vi "Save DataBuffer.vi"(0 "File Parameter":T8={"Filename Prefix"="MyData", "Extension"=enum."±Field", "Suffix"="", "Current Path"=path "/opticsmac/Users/Data"}, 7 "User Comments":string="This data's for you!\nType \u0011-H to get a help window for the various controls.", 13 "FileFormat":T7={"File Format"=enum."Macintosh (EOL: CR)", "Delimiter"=enum."TAB", "SaveComments?"=enum."Saved in the Header Area"}) -> (4 "File Info output":T1={"FilePath"=path "/DATA/Labview Items", "Field (T)"=55.0, "Temperature (K)"=77.0, "X-Axis"=enum."nm", "Center nm"=55.0, "Current Grating Density"=enum."600", "CCD Parameters"={"Exposure Time (s)"=0.2, "Offset"=0.0, "BkgrdCrct"=FALSE, "Shutter"=FALSE, "Mode"=enum."Regular", "Repetition"=4, "dt or s"=0.0}, "Operation Mode"=enum."NML Data Acquisition", "Exp Index"=0, "Index_repetition"=0, "Index"=0, "Current Detector"=enum."CCD-1024x256"} {"CCD Parameters"."dt or s" format="%#.6f"; "CCD Parameters"."Repetition" min=1; "CCD Parameters"."Offset" format="%#.2f"; "CCD Parameters"."Exposure Time (s)" min=0.02 max=6000.0 format="%#.2f"; "Center nm" format="%.2f"; "Temperature (K)" format="%.2f"; "Field (T)" format="%.2f"})   [LabVIEW 2019]
doc: "Write (FIFO) or retrieve (LIFO) data from the buffer.\n\nWhen write to the buffer, set the desired \"Buffer Size\" and run the VI several iterations. Notice that initially, the buffer grows to reach \"Buffer Size\" and then the input data flows from the last buffer element through to the zero element on each iteration (First In, First Out).\n\nWhen read from the buffer, set the Read# to the nth previous input data, i.e. counting reversely, with the most recent input counted as the 1st readout. If the input is out of current buffer size, an error is returned. (Last In, First Out)"
uses:
  Globals and TypeDefs/Type Definitions.llb/FilePathParameter.ctt
  Globals and TypeDefs/Type Definitions.llb/FileFormatParameter.ctt
  Globals and TypeDefs/Type Definitions.llb/FileInfoParameter.ctt
  Globals and TypeDefs/Type Definitions.llb/Wavelength Unit.ctt
  Globals and TypeDefs/Type Definitions.llb/McPherson Grating Density.ctl
  Globals and TypeDefs/Type Definitions.llb/CCDParameter.ctt
  Globals and TypeDefs/Type Definitions.llb/OperationMode.ctt
  Globals and TypeDefs/Type Definitions.llb/ListOfDetectors.ctt
  File and save/X-Axis_Generator_morph.vi
panel:
  out "X-Axis":i32(ring)=1 items=["Point #", "nm", "eV", "meV", "cm-1"]
  in  "continue2":bool=TRUE
  in  "Speed":u16(slide)=100 min=50 max=5000 step=50 scale=10.0..5000.0
  in  "Movie":bool
  out "Continue?":bool
  out "File Contents":string
  in  "WL unit":i32(ring)=1 items=["Wavelength", "nm", "eV", "meV", "cm-1"]
  in  "Save":bool
  in  "Cancel":bool
  out "File Path":path
  out "?":T9(graph)
  in  "Read#":u16(slide)=1 min=1 max=27 step=1 scale=1.0..27.0
  # "Latest"
  # "Erliest"
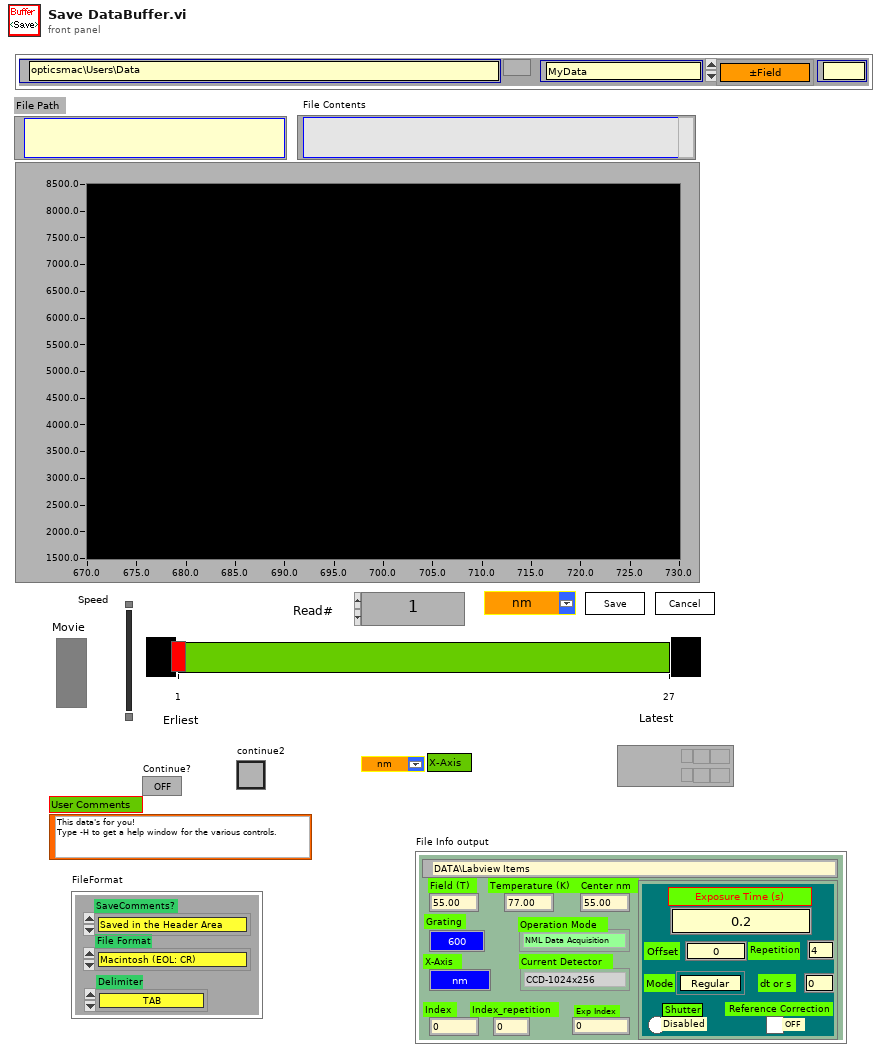
[diagram p1: front panel]
types:
  T1 = typedef "FileInfoParameter.ctt" = cluster{"FilePath":path, "Field (T)":dbl, "Temperature (K)":dbl, "X-Axis":T2, "Center nm":dbl, "Current Grating Density":T3, "CCD Parameters":T4, "Operation Mode":T5, "Exp Index":u32, "Index_repetition":u16, "Index":u16, "Current Detector":T6}
  T2 = typedef "Wavelength Unit.ctt" = enum8{"Point", "nm", "eV", "meV", "cm_1"}
  T3 = typedef "McPherson Grating Density.ctl" = enum8{"150", "300", "600", "1200", "1800"}
  T4 = typedef "CCDParameter.ctt" = cluster{"Exposure Time (s)":dbl, "Offset":dbl, "BkgrdCrct":bool, "Shutter":bool, "Mode":enum8{"Regular", "OverExp Cor", "SpikeRemove", "ForCalibration"}, "Repetition":u16, "dt or s":dbl}
  T5 = typedef "OperationMode.ctt" = enum16{"Standby", "CCD Single Shot", "CCD Sequence Shots", "CCD Custom Shots", "CCD Reference Shot", "Step Scanning ", "Time Scanning", "NML Data Acquisition"}
  T6 = typedef "ListOfDetectors.ctt" = enum8{"CCD-1024x256", "InGaAs PDA-1024x1", "CCD-1340x400", "Ge Single Channel", "Si Single Channel", "PMT Single Channel"}
  T7 = typedef "FileFormatParameter.ctt" = cluster{"File Format":enum16{"Macintosh (EOL: CR)", "Unix (EOL: LF)", "DOS/Windows (EOL: CR+LF)"}, "Delimiter":enum16{"TAB", "COMMA", "SPACE"}, "SaveComments?":enum16{"Bare data only", "Saved in the Header Area", "Saved as a Parameter File"}}
  T8 = typedef "FilePathParameter.ctt" = cluster{"Filename Prefix":string, "Extension":enum16{"none", "\".001\",\".002\", ...", "001 (No dot)", "±Field", "pField nField", "Temperature", "Wavelength", "T(K)±H(T)", "(nm)T(K)±H(T)", "User Defined"}, "Suffix":string, "Current Path":path}
  T9 = cluster{"Ramp Pattern":dbl[], "Sinc Pattern":dbl[]}
  T10 = enum16{"Pass", "Write", "Read", "ReadPlotBlock", "Initialize", "InitFromBufferInput", "Resize Buffer"}
  T11 = enum16{"open", "open or create", "create or replace", "create", "open (read only)"}
  T12 = enum16{"Auto Data Saving", "Manual Data Saving", "Auto Sequence Saving", "Sequence Saving from Data Buffer"}
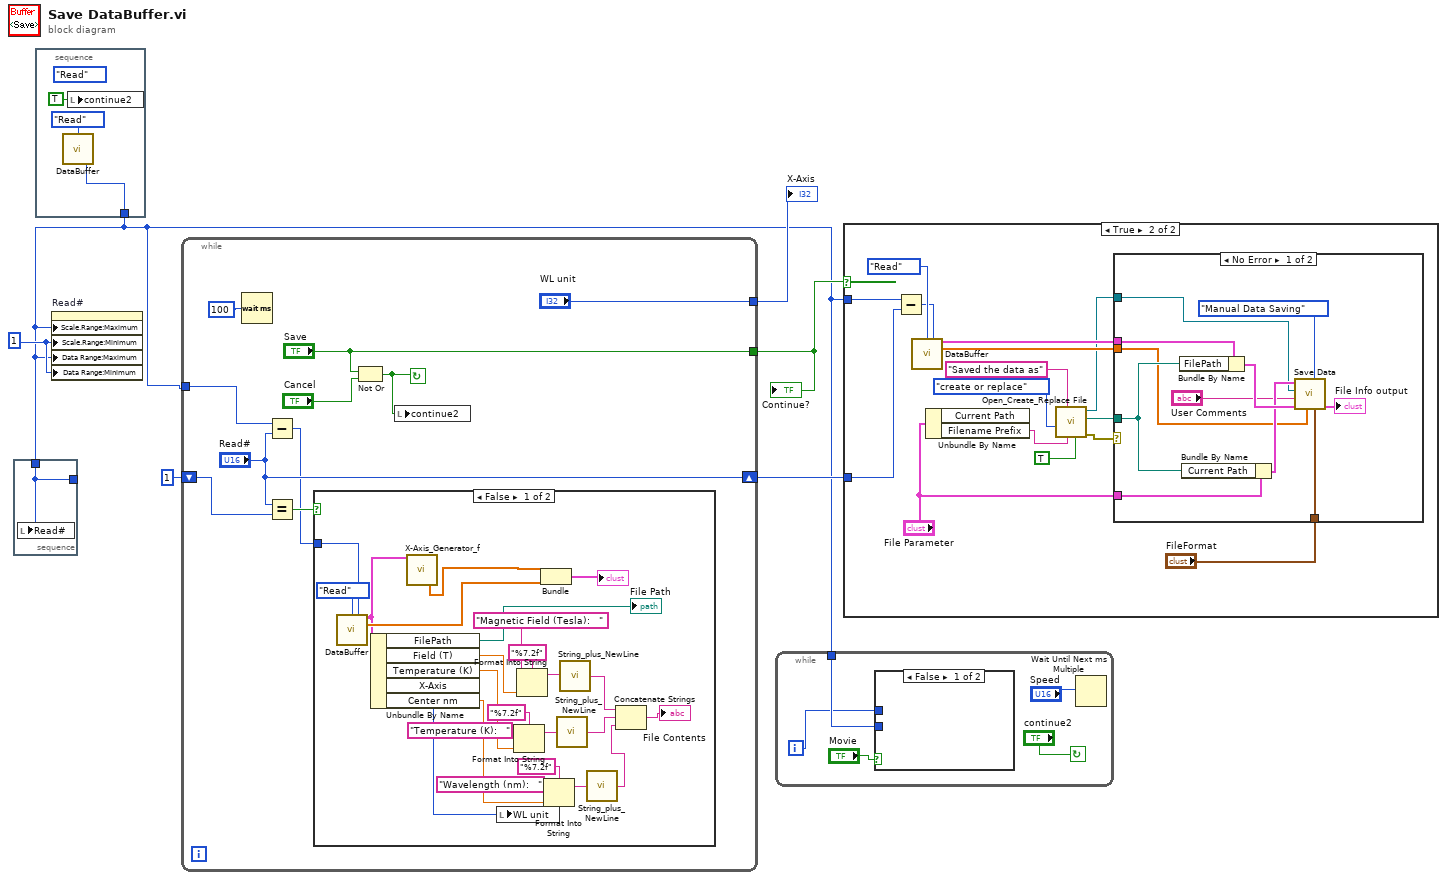
[diagram p0: block diagram]
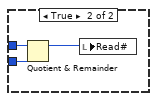
[diagram p5: hidden frame]
diagram:
  w5 = u32 1 ("milliseconds to wait")
  n1 = stacked-sequence {
    tunnel: [w8] -> w1
    frame #0 {
      (unwired) enum16{"Pass", "Write", "Read", "Initialize"}."Read" ("Action")
      n2 = call "DataBuffer.vi"("Action"=T10."Read") -> ("Current Buffer Size"=w8:i32)  [unwired: 10 in, 4 out]
      n3 = local write "continue2"(TRUE ("Boolean")) -> ()
    }
  }
  n4 = stacked-sequence {
    tunnel: w1 -> [w10]
    tunnel: [w10] -> _
    frame #0 {
      n5 = local write "Read#"(w10) -> ()
    }
  }
  n6 = property on="Read#" class="Slide (strict)"("Scale.Range:Maximum"=w1, "Scale.Range:Minimum"=w5, "Data Range:Maximum"=w1, "Data Range:Minimum"=w5) -> ()  [unwired: 2 in, 2 out]
  n7 = while {
    tunnel: w1 -> [w15]
    shift-left: u8 1 ("Read#") -> [w17]
    shift-right: ["Read#"] -> w2
    tunnel: ["Save"] -> w3
    tunnel: ["WL unit"] -> w4
    stop <- w12 continue-if-true
    n8 = Wait (ms)(milliseconds to wait=u32 100) -> ()  [unwired: 1 out]
    n9 = Subtract(x=w15, y="Read#") -> (x-y=w13:i32)
    n10 = Equal?(x="Read#", y=w17) -> (x = y?=w16:bool)
    n11 = case shown="False" w16 {
      tunnel: w13 -> [w34 _]
      frame False {
        n12 = call "DataBuffer.vi"("Action"=T10."Read", "Read#"=w34) -> ("File Info Out"=w31:T1, "Y Array out"=w32:dbl[])  [unwired: 9 in, 3 out]
        n13 = Unbundle By Name(w31) -> ("FilePath"=→"File Path":path, "Field (T)"=w29:dbl, "Temperature (K)"=w28:dbl, "X-Axis"=w27:T2, "Center nm"=w22:dbl)
        n14 = call-poly "X-Axis_Generator_f.vi"("File Info In"=w31) -> ("X-axis"=w33:dbl[])  [unwired: 11 in, 7 out]
        n15 = local write "WL unit"(w27) -> ()
        n16 = Format Into String(format string="%7.2f", initial string="Temperature (K):   ", w28) -> (resulting string=w40:string)  [unwired: 1 in, 1 out]
        n17 = Format Into String(format string="%7.2f", initial string="Magnetic Field (Tesla):   ", w29) -> (resulting string=w42:string)  [unwired: 1 in, 1 out]
        n18 = Bundle("X-axis"=w33, "Y Array out"=w32) -> (→"?":cluster{"X-axis":dbl[], "Y Array out":dbl[]})  [unwired: 1 in]
        n19 = Format Into String(format string="%7.2f", initial string="Wavelength (nm):   ", w22) -> (resulting string=w25:string)  [unwired: 1 in, 1 out]
        n20 = call "String_plus_NewLine.vi"("Input String"=w40) -> ("Input String +[\\n]"=w36:string)
        n21 = call "String_plus_NewLine.vi"("Input String"=w42) -> ("Input String +[\\n]"=w37:string)
        n22 = call "String_plus_NewLine.vi"("Input String"=w25) -> ("Input String +[\\n]"=w21:string)
        n23 = Concatenate Strings(w37, w36, w21) -> (→"File Contents":string)
      }
      frame True {
      }
    }
    n24 = Not Or(1:"Cancel", 2:"Save") -> (0:w12:bool)
    n25 = local write "continue2"(w12) -> ()
  }
  "Continue?" <- w3
  "X-Axis" <- w4
  n26 = while {
    tunnel: w1 -> [w49]
    i -> [w46]
    stop <- "continue2" continue-if-true
    n27 = case shown="False" "Movie" {
      tunnel: w49 -> [_ w52]
      tunnel: w46 -> [_ w50]
      frame False {
      }
      frame True {
        n28 = Quotient & Remainder(x=w50, y=w52) -> (x-y*floor(x/y)=w51:i32)  [unwired: 1 out]
        n29 = local write "Read#"(w51) -> ()
      }
    }
    n30 = Wait Until Next ms Multiple(millisecond multiple="Speed") -> ()  [unwired: 1 out]
  }
  n31 = case shown="True" w3 {
    tunnel: w2 -> [_ w54]
    tunnel: w1 -> [_ w55]
    frame False {
    }
    frame True {
      n32 = Subtract(x=w55, y=w54) -> (x-y=w53:i32)
      n33 = call "DataBuffer.vi"("Action"=T10."Read", "Read#"=w53) -> ("File Info Out"=w64:T1, "Y Array out"=w61:dbl[])  [unwired: 9 in, 3 out]
      n34 = Unbundle By Name("File Parameter") -> ("Filename Prefix"=w65:string)  [unwired: 1 out]
      n35 = call <vilib>:"Open_Create_Replace File.vi"("advisory dialog? (display:T)"=TRUE, "default name"=w65, "prompt"="Saved the data as", "function (open:0)"=T11."create or replace") -> ("error out"=w59:errorcluster, "new file path"=w62:path, "refnum"=w56:refnum<file>)  [unwired: 4 in, 1 out]
      n36 = case shown="No Error" w59 {
        tunnel: w64 -> [w78 _]
        tunnel: "File Parameter" -> [w75 _]
        tunnel: w62 -> [w74 _]
        tunnel: w61 -> [w71 _]
        tunnel: "FileFormat" -> [w70 _]
        tunnel: w56 -> [w68 _]
        frame No Error {
          n37 = Bundle By Name(cluster=w78, "FilePath"=w74) -> (w77:T1)
          n38 = Bundle By Name(cluster=w75, "Current Path"=w74) -> (w73:T8)
          n39 = call "Save Data.vi"("FileFormat"=w70, "Saving Mode"=T12."Manual Data Saving", "Data"=w71, "File Info Input"=w77, "User Comments"="User Comments", "File Refnum"=w68, "File Parameter"=w73) -> ("File Info output"=→"File Info output":T1)  [unwired: 4 in]
        }
        frame Error {
        }
      }
    }
  }
